vi "ReadIntensity.vi"(8 "Lookup":u32[](array[numeric]), 9 "IntenOff":u32, 10 "IntensityHead":T1, 11 "RefIn":refnum<file>) -> (2 "Intensity":u16[][](array[numeric]), 3 "IntenPic":picture, 4 "RefOut":refnum<file>)   [LabVIEW 2012]
uses:
  ImageHeaderType.ctl
  <vilib>/picture/picture.llb/Draw 8-Bit Pixmap.vi
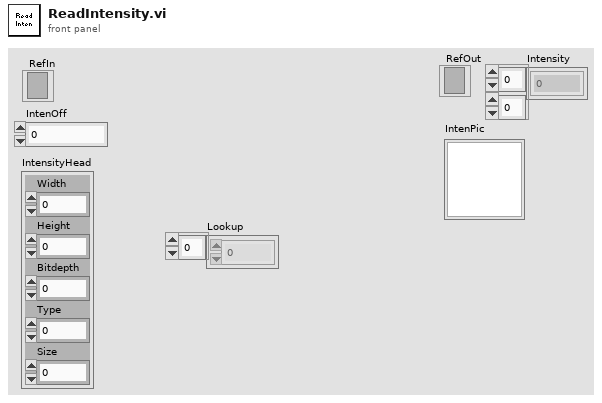
[diagram p1: front panel]
types:
  T1 = typedef "ImageHeaderType.ctl" = cluster{"Width":u32, "Height":u32, "Bitdepth":u32, "Type":u32, "Size":u32}
  T2 = enum16{"big-endian, network order", "native, host order", "little-endian"}
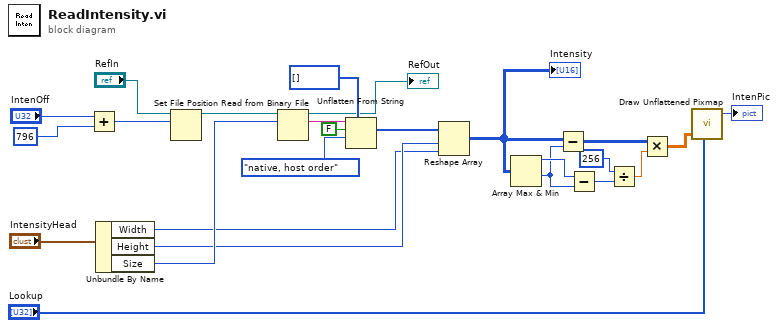
[diagram p0: block diagram]
diagram:
  n1 = Add(x="IntenOff", y=u32 796) -> (x+y=w15:u32)
  n2 = Unbundle By Name("IntensityHead") -> ("Width"=w9:u32, "Height"=w10:u32, "Size"=w13:u32)
  n3 = Set File Position(offset (in bytes) (0)=w15, refnum="RefIn") -> (refnum out=w21:refnum<file>)  [unwired: 2 in, 1 out]
  n4 = Read from Binary File(10:w13, 11:w21) -> (2:w22:string, 3:→"RefOut":refnum<file>)  [unwired: 4 in, 2 out]
  n5 = Unflatten From String(type=u16[] [], binary string=w22, data includes array or string size? (T)=FALSE, byte order (0:big-endian, network order)=T2."native, host order") -> (value=w20:u16[])  [unwired: 1 in, 2 out]
  n6 = Reshape Array(w20, w10, w9) -> (w2:u16[][])
  "Intensity" <- w2
  n7 = Array Max & Min(array=w2) -> (max value=w8:u16, min value=w7:u16)  [unwired: 2 out]
  n8 = Subtract(x=w2, y=w7) -> (x-y=w3:u16[][])
  n9 = Subtract(x=w8, y=w7) -> (x-y=w6:u16)
  n10 = Divide(x=256, y=w6) -> (x/y=w4:dbl)
  n11 = Multiply(x=w3, y=w4) -> (x*y=w1:dbl[][])
  n12 = call-poly <vilib>:"Draw Unflattened Pixmap.vi"("data"=w1, "color table"="Lookup") -> ("new picture"=→"IntenPic":picture)  [unwired: 7 in]
